vi "Generic command handler.vi"(8 "error in (no error)":errorcluster, 10 "Message in":refnum<class "GenericMessage.lvclass">, 11 "ImageStack in":refnum<class "Invivo_ImageStack.lvclass">) -> (0 "error out":errorcluster, 2 "value":string, 3 "ImageStack out":refnum<class "Invivo_ImageStack.lvclass">)   [LabVIEW 2012, in "Invivo_ImageStack.lvclass"]
doc: "The generic_command_handler processes the command 'generic'. Commands which are not part of the predefined list of commands fall under the 'generic' command for special activity."
uses:
  Invivo_ImageStack.lvclass
  <vilib>/Distrio/Murmex/GenericMessage/GenericMessage.lvclass
  <vilib>/Distrio/Murmex/Murmex/Murmex.lvclass
  Invivo_ImageStack.lvclass/Invivo_ImageStack.ctl
  <vilib>/Distrio/Murmex/Message/Message.lvclass
panel:
  # "This method is called when the GENERIC\ntrigger is sent. \n\nOverride this method when your component needs to\nrespond to this trigger. \n\nCall parent for proper implementation"
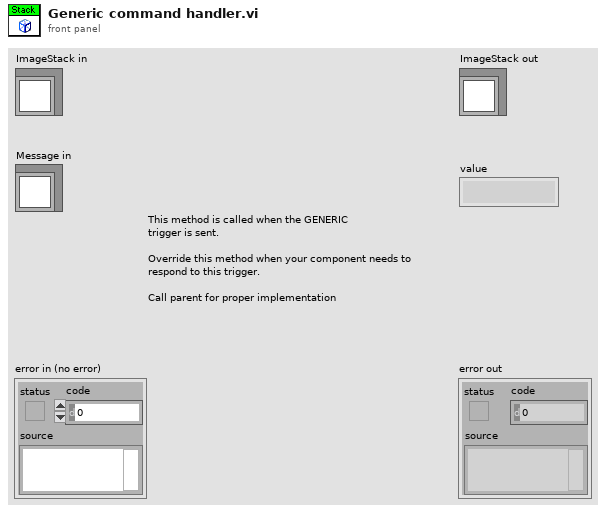
[diagram p1: front panel]
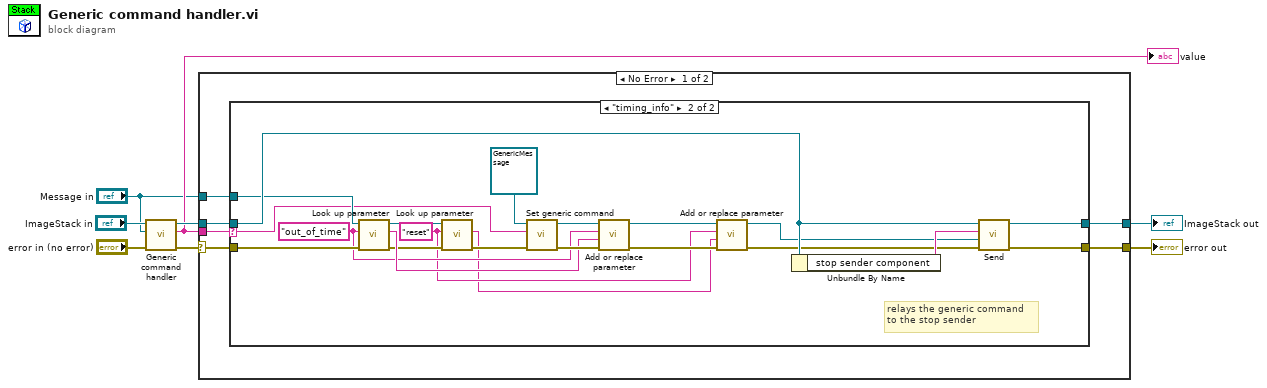
[diagram p0: block diagram]
diagram:
  n1 = call-parent "Generic command handler.vi"("error in (no error)"="error in (no error)", "Message in"="Message in", "Murmex in"="ImageStack in") -> ("error out"=w6:errorcluster, "value"=w2:string, "Murmex out"=w5:refnum<class "Invivo_ImageStack.lvclass">)  [unwired: 6 in]
  "value" <- w2
  n2 = case shown="No Error" w6 {
    selector: w6 -> [w12 w38]
    tunnel: w5 -> [w13 w39]
    tunnel: w2 -> [w14 _]
    tunnel: [w11 w39] -> w4
    tunnel: [w10 w38] -> w3
    tunnel: "Message in" -> [w9 _]
    frame No Error {
      n3 = case shown="\"timing_info\"" w14 {
        selector: w14 -> [_ w29]
        tunnel: w13 -> [w16 w34]
        tunnel: w12 -> [w15 w33]
        tunnel: [w16 w37] -> w11
        tunnel: [w15 w36] -> w10
        tunnel: w9 -> [_ w32]
        frame Default {
        }
        frame "timing_info" {
          w18 = "reset" ("name")
          w26 = "out_of_time" ("name")
          # "relays the generic command\nto the stop sender"
          n4 = call <vilib>:"Look up parameter.vi"("error in (no error)"=w33, "name"=w26, "Message in"=w32) -> ("error out"=w21:errorcluster, "key"=w27:string, "Message out"=w19:refnum<class "GenericMessage.lvclass">)  [unwired: 5 in, 1 out]
          n5 = call <vilib>:"Look up parameter.vi"("error in (no error)"=w21, "name"=w18, "Message in"=w19) -> ("error out"=w20:errorcluster, "key"=w17:string)  [unwired: 5 in, 2 out]
          n6 = call <vilib>:"Set generic command.vi"("error in (no error)"=w20, "generic command"=w29, "GenericMessage in"=refnum<class "GenericMessage.lvclass"> refnum ("Distrio Murmex 1.2:GenericMessage")) -> ("error out"=w31:errorcluster, "GenericMessage out"=w28:refnum<class "GenericMessage.lvclass">)  [unwired: 7 in]
          n7 = call <vilib>:"Add or replace parameter.vi"("error in (no error)"=w31, "value"=w27, "name"=w26, "Message in"=w28) -> ("error out"=w25:errorcluster, "Message out"=w24:refnum<class "GenericMessage.lvclass">)  [unwired: 6 in]
          n8 = call <vilib>:"Add or replace parameter.vi"("error in (no error)"=w25, "value"=w17, "name"=w18, "Message in"=w24) -> ("error out"=w22:errorcluster, "Message out"=w23:refnum<class "GenericMessage.lvclass">)  [unwired: 6 in]
          n9 = Unbundle By Name(w34) -> ("stop sender component"=w35:string)
          n10 = call <vilib>:"Send.vi"("error in (no error)"=w22, "Message"=w23, "recipient"=w35, "Murmex in"=w34) -> ("error out"=w36:errorcluster, "Murmex out"=w37:refnum<class "Invivo_ImageStack.lvclass">)  [unwired: 6 in]
        }
      }
    }
    frame Error {
    }
  }
  "error out" <- w3
  "ImageStack out" <- w4
